vi "CC Script Parse Define Dithering.vi"(8 "error in (no error)":errorcluster, 9 "To Script?":bool, 10 "Dithering Offsets in":T1, 11 "DefineDithering Parameters":string="\"Dithering Test Parse\" (1,2),(2,4),(3,5)") -> (0 "error out":errorcluster, 2 "Dithering Offsets out":T1, 3 "Script out":string="ObjectName \"RA\":\"123.456\",\"DEC\":\"4546.54\"")   [LabVIEW 2021]
uses:
  typedefs/CC cluster Offset Dithering.ctl
  typedefs/CC Dithering Offsets.ctl
  <vilib>/regexp/Match Regular Expression.xnode
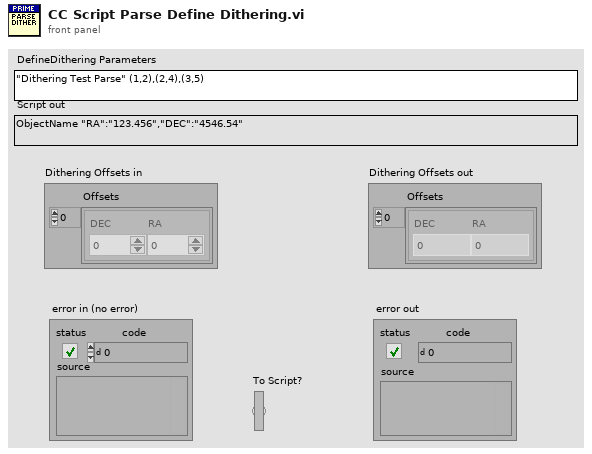
[diagram p1: front panel]
types:
  T1 = typedef "CC cluster Offset Dithering.ctl" = cluster{"Offsets":T2[]}
  T2 = typedef "CC Dithering Offsets.ctl" = cluster{"DEC":dbl, "RA":dbl}
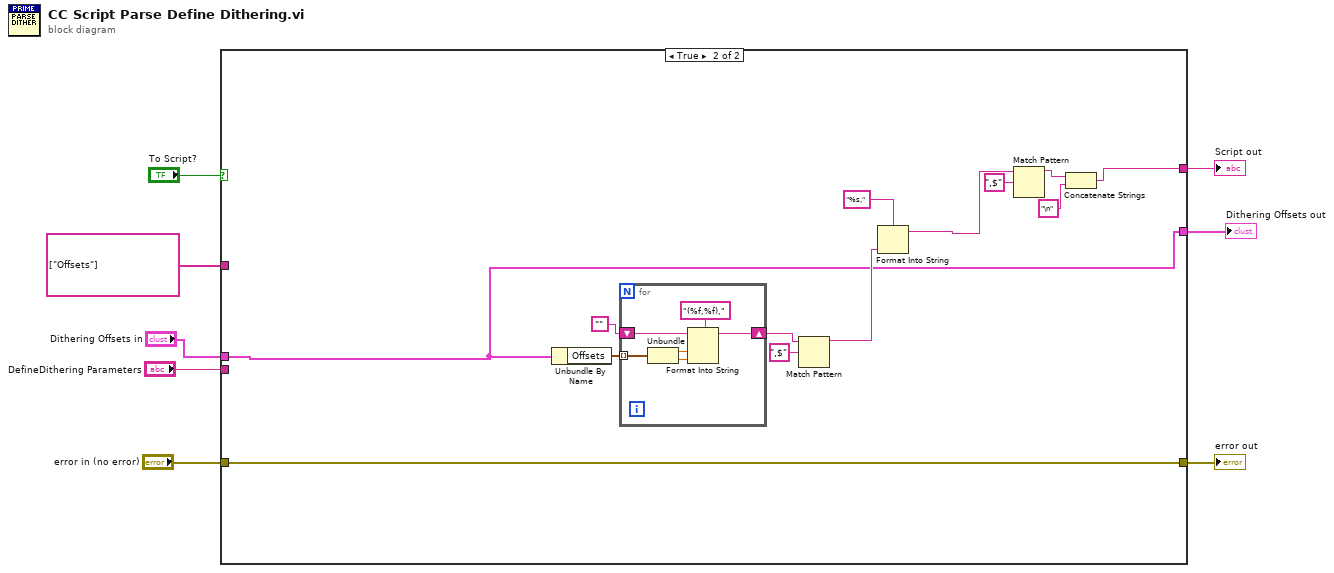
[diagram p0: block diagram]
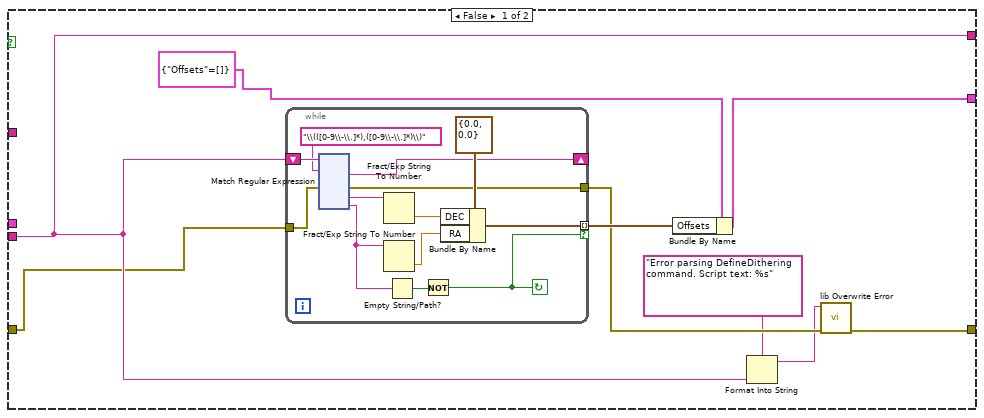
[diagram p2: hidden frame]
diagram:
  n1 = case shown="True" "To Script?" {
    tunnel: "DefineDithering Parameters" -> [w10 _]
    tunnel: string[] ["Offsets"] -> [_ _]
    tunnel: [w17 w151] -> w1
    tunnel: "error in (no error)" -> [w9 w158]
    tunnel: [w15 w158] -> w5
    tunnel: "Dithering Offsets in" -> [_ w151]
    tunnel: [w10 w159] -> w2
    frame False {
      n2 = while {
        shift-right: [w23] -> _
        shift-left: w10 -> [w30]
        tunnel: w9 -> [w28]
        tunnel: [w22] -> w16 mode=indexing if=w19
        tunnel: [w18] -> w14
        stop <- w19 continue-if-true
        n3 = xnode "Match Regular Expression"("input string"=w30, "regular expression"="\\(([0-9\\-\\.]*),([0-9\\-\\.]*)\\)", "error in"=w28) -> ("after match"=w23:string, "error out"=w18:errorcluster, "submatch 1"=w27:string, "submatch 2"=w21:string)  [unwired: 3 in, 3 out]
        n4 = Fract/Exp String To Number(string=w27) -> (number=w25:dbl)  [unwired: 3 in, 1 out]
        n5 = Fract/Exp String To Number(string=w21) -> (number=w24:dbl)  [unwired: 3 in, 1 out]
        n6 = Empty String/Path?(string/path=w21) -> (empty?=w20:bool)
        n7 = Not(x=w20) -> (.not. x?=w19:bool)
        n8 = Bundle By Name(cluster=T2 {"DEC"=0.0, "RA"=0.0} ("Dither Offsets"), "DEC"=w25, "RA"=w24) -> (w22:T2)
      }
      n9 = Bundle By Name(cluster=T1 {"Offsets"=[]} ("Dithering Offsets"), "Offsets"=w16) -> (w17:T1)
      n10 = Format Into String(format string="Error parsing DefineDithering command. Script text: %s", w10) -> (resulting string=w12:string)  [unwired: 2 in, 1 out]
      n11 = call "lib Overwrite Error.vi"("error in (no error)"=w14, "Error Message"=w12) -> ("error out"=w15:errorcluster)  [unwired: 9 in]
    }
    frame True {
      n12 = Unbundle By Name(w151) -> ("Offsets"=w154:T2[])
      n13 = for {
        shift-right: [w167] -> w152
        shift-left: "" -> [w168]
        tunnel: w154 -> [w166] mode=indexing
        n14 = Unbundle(w166) -> ("DEC"=w164:dbl, "RA"=w165:dbl)
        n15 = Format Into String(format string="(%f,%f),", initial string=w168, w164, w165) -> (resulting string=w167:string)  [unwired: 1 in, 1 out]
      }
      n16 = Match Pattern(string=w152, regular expression=",$") -> (before substring=w156:string)  [unwired: 1 in, 3 out]
      n17 = Format Into String(format string="%s,", w156) -> (resulting string=w163:string)  [unwired: 2 in, 1 out]
      n18 = Match Pattern(string=w163, regular expression=",$") -> (before substring=w161:string)  [unwired: 1 in, 3 out]
      n19 = Concatenate Strings(w161, "\n" ("string")) -> (w159:string)
    }
  }
  "error out" <- w5
  "Dithering Offsets out" <- w1
  "Script out" <- w2
